vi "remove zero from page.vi"(6 "page number":i32, 11 "Cycle data by seq":dbl[][][](array[numeric])) -> (3 "array w/ subset deleted":dbl[][](array[numeric]))   [LabVIEW 2016]
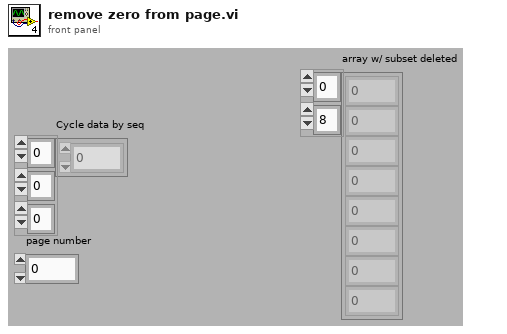
[diagram p1: front panel]
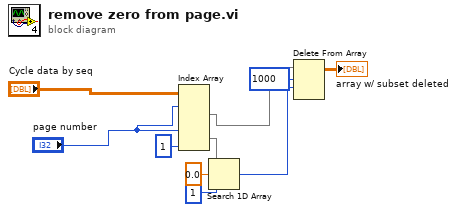
[diagram p0: block diagram]
diagram:
  n1 = Index Array(array="Cycle data by seq", index (dim 0) #1="page number", index (dim 0) #2="page number", index (dim 2) #2=1 ("disabled index (col)")) -> (element #1=w4:dbl[][], element #2=w9:dbl[])  [unwired: 3 in]
  n2 = Search 1D Array(1D array=w9, element=0.0, start index (0)=1) -> (index of element=w1:i32)
  n3 = Delete From Array(array=w4, length=1000, index (row)=w1) -> (array with subset deleted=→"array w/ subset deleted":dbl[][])  [unwired: 1 in, 1 out]
